vi "SPC_get_FPGA_Version.vi"(8 "Error In":errorcluster, 10 "Module No":i16, 11 "DLL Path":path) -> (0 "Error Out":errorcluster, 2 "Module No":i16, 3 "DLL Path":path, 4 "FPGA Version":i32)   [LabVIEW 2023]
doc: "This function reads out the current installed FPGA version of the used SPC card in decimal.\n\nJuly 2020\nFrank Quadt\ninfo@becker-hickl.com"
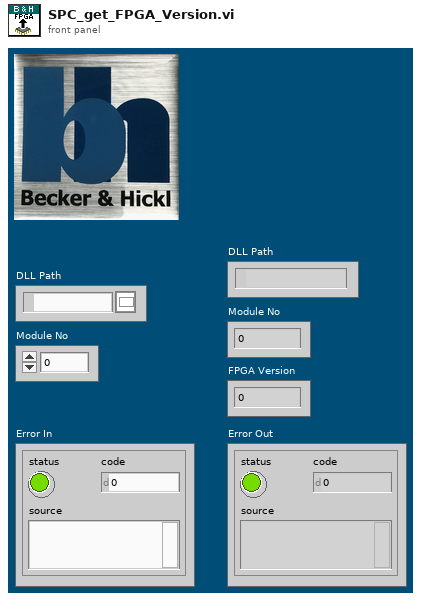
[diagram p1: front panel]
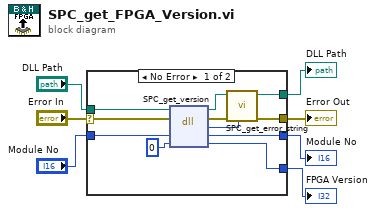
[diagram p0: block diagram]
diagram:
  n1 = case shown="No Error" "Error In" {
    selector: "Error In" -> [w17 w19]
    tunnel: "DLL Path" -> [w18 w21]
    tunnel: [w14 w19] -> w5
    tunnel: [w13 w20] -> w4
    tunnel: [w11 w21] -> w3
    tunnel: "Module No" -> [w10 w20]
    tunnel: [w8 _] -> w1
    frame No Error {
      n2 = dll-call lib="C:/Program Files (x86)/BH/SPCM/DLL/spcm64.dll" fn="SPC_get_version"(path in=w18, error in=w17, "Module No"=w10, "FPGA Version"=0) -> (path out=w16:path, error out=w15:errorcluster, "return type"=w12:i16, "Module No"=w13:i16, "FPGA Version"=w8:i32)  [unwired: 1 in]
      n3 = call "SPC_get_error_string.vi"("ErrorID"=w12, "Error In"=w15, "DLL Path"=w16) -> ("Error Out"=w14:errorcluster, "DLL Path"=w11:path)  [unwired: 6 in, 1 out]
    }
    frame Error {
    }
  }
  "Error Out" <- w5
  "Module No" <- w4
  "DLL Path" <- w3
  "FPGA Version" <- w1
